vi "tp.vi"() -> ()   [LabVIEW 2017]
panel:
  out "Modified Array Out":dbl[](array[numeric])=[2.0]
  in  "1/0_array":dbl[](array[numeric])
  in  "input array":dbl[](array[numeric])
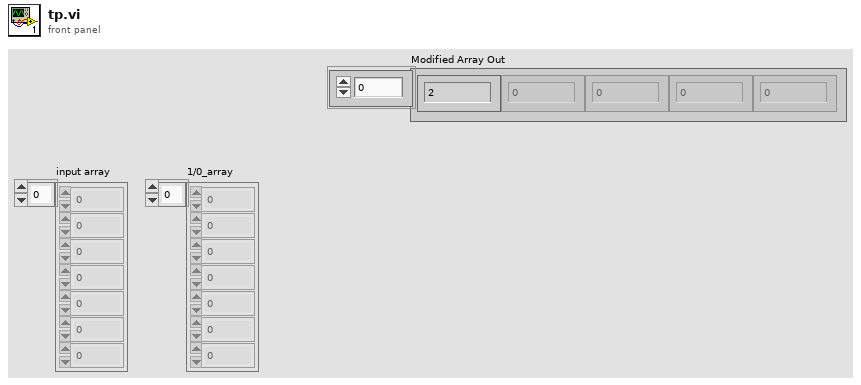
[diagram p1: front panel]
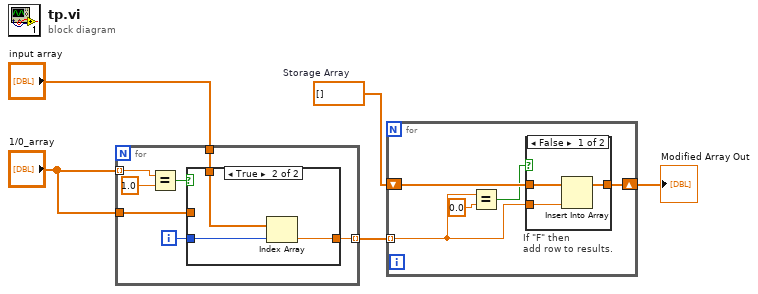
[diagram p0: block diagram]
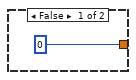
[diagram p3: hidden frame]
diagram:
  w3 = dbl[] []  # Storage Array
  n1 = for {
    tunnel: "1/0_array" -> [w12] mode=indexing
    tunnel: "1/0_array" -> [w9]
    tunnel: "input array" -> [w8]
    tunnel: [w6] -> w1 mode=indexing
    i -> [w7]
    n2 = Equal?(x=w12, y=1.0) -> (x = y?=w10:bool)
    n3 = case shown="True" w10 {
      tunnel: w9 -> [_ _]
      tunnel: w8 -> [_ w16]
      tunnel: w7 -> [_ w15]
      tunnel: [0 w14] -> w6
      frame False {
      }
      frame True {
        n4 = Index Array(array=w16, index=w15) -> (element=w14:dbl)
      }
    }
  }
  n5 = for {
    tunnel: w1 -> [w19] mode=indexing
    shift-right: [w20] -> w2
    shift-left: w3 -> [w21]
    n6 = Equal?(x=w19, y=0.0) -> (x = y?=w17:bool)
    n7 = case "If \"F\" then \nadd row to results." shown="False" w17 {
      tunnel: w21 -> [w24 w25]
      tunnel: w19 -> [w23 _]
      tunnel: [w22 w25] -> w20
      frame False {
        n8 = Insert Into Array(array=w24, new element=w23) -> (w22:dbl[])  [unwired: 1 in]
      }
      frame True {
      }
    }
  }
  "Modified Array Out" <- w2
